vi "Static Test.vi"(5 "Mechanical Zero":dbl, 9 "read buffer":string) -> (4 "Elbow Angle (deg)":dbl, 6 "Goniometer\nAngle Raw":dynamicdata(graph), 8 "Static LF":dbl, 10 "Static Load Force":dynamicdata(graph), 14 "Grip Force":dynamicdata(graph), 15 "GF":dbl)   [LabVIEW 2018]
doc: "VI for GF and LF conversion."
panel:
  out "Dynamic Load Force":dbl
  # "\"Throw away\" data"
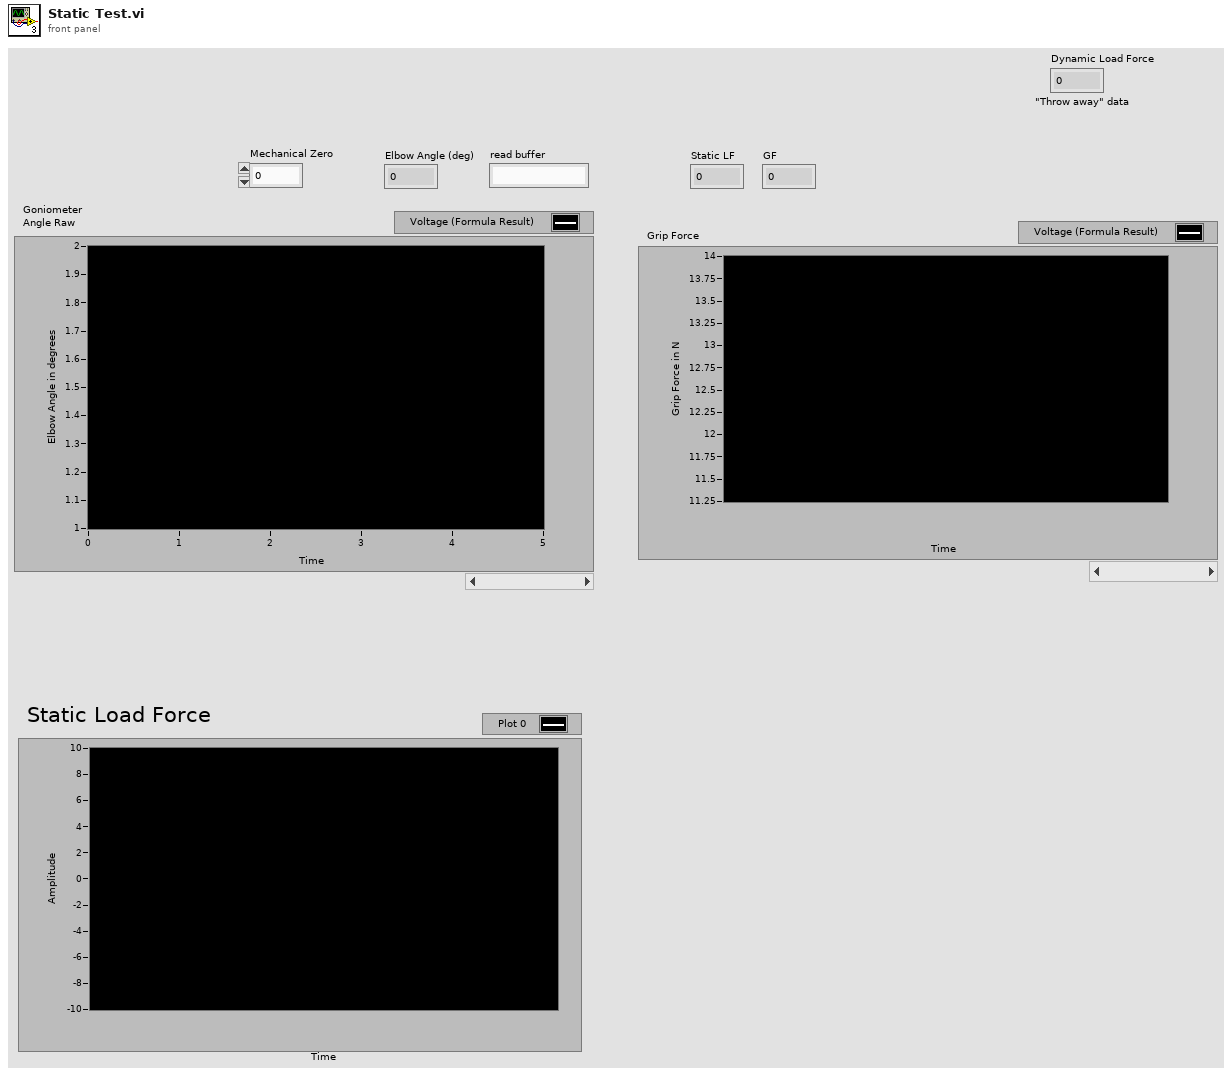
[diagram p1: front panel]
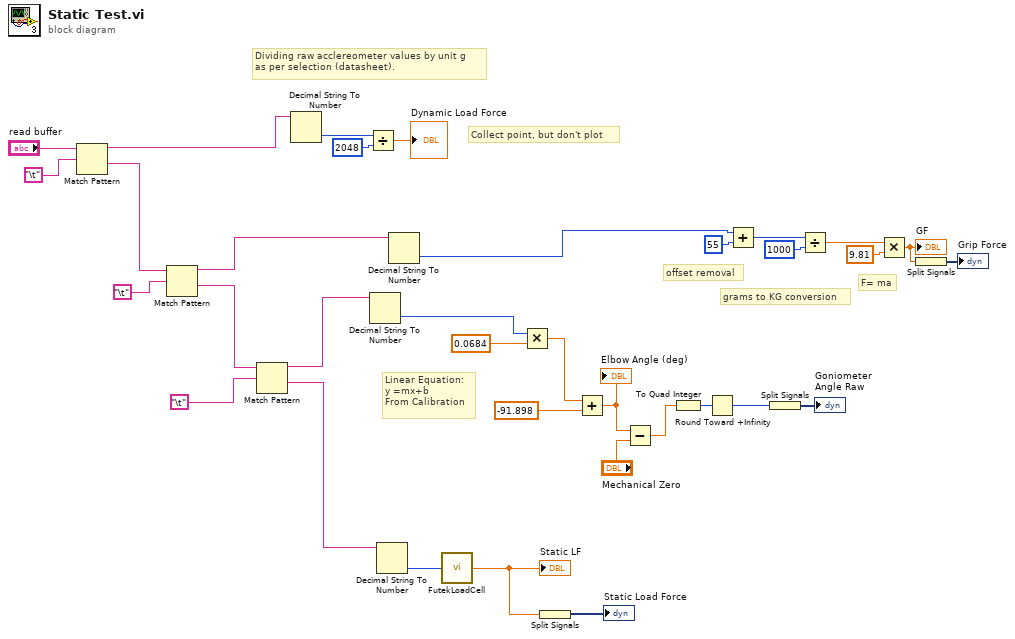
[diagram p0: block diagram]
diagram:
  # "Collect point, but don't plot"
  # "F= ma"
  # "offset removal"
  # "grams to KG conversion"
  # "Linear Equation:\ny =mx+b\nFrom Calibration"
  # "Dividing raw acclereometer values by unit g\nas per selection (datasheet)."
  n1 = Match Pattern(string="read buffer", regular expression="\t") -> (before substring=w34:string, after substring=w28:string)  [unwired: 1 in, 2 out]
  n2 = Match Pattern(string=w28, regular expression="\t") -> (before substring=w27:string, after substring=w16:string)  [unwired: 1 in, 2 out]
  n3 = Match Pattern(string=w16, regular expression="\t") -> (before substring=w15:string, after substring=w14:string)  [unwired: 1 in, 2 out]
  n4 = Decimal String To Number(string=w34) -> (number=w31:i32)  [unwired: 2 in, 1 out]
  n5 = Divide(x=w31, y=2048) -> (x/y=→"Dynamic Load Force":dbl)
  n6 = Decimal String To Number(string=w15) -> (number=w22:i32)  [unwired: 2 in, 1 out]
  n7 = Decimal String To Number(string=w14) -> (number=w2:i32)  [unwired: 2 in, 1 out]
  n8 = Decimal String To Number(string=w27) -> (number=w4:i32)  [unwired: 2 in, 1 out]
  n9 = call "FutekLoadCell.vi"("Futek Sensor Reading"=w2) -> ("Futek Force"=w1:dbl)
  "Static LF" <- w1
  n10 = Multiply(x=w22, y=0.0684 ("x")) -> (x*y=w25:dbl)
  n11 = Split Signals(w1) -> (→"Static Load Force":dynamicdata)  [unwired: 1 in]
  n12 = Add(x=w25, y=-91.898 ("x")) -> (x+y=w20:dbl)
  "Elbow Angle (deg)" <- w20
  n13 = Subtract(x=w20, y="Mechanical Zero") -> (x-y=w21:dbl)
  n14 = To Quad Integer(1:w21) -> (0:w18:i64)
  n15 = Round Toward +Infinity(x=w18) -> (ceil(x): smallest int >= x=w17:i64)
  n16 = Add(x=w4, y=55) -> (x+y=w10:i32)
  n17 = Split Signals(w17) -> (→"Goniometer\nAngle Raw":dynamicdata)  [unwired: 1 in]
  n18 = Divide(x=w10, y=1000) -> (x/y=w7:dbl)
  n19 = Multiply(x=w7, y=9.81) -> (x*y=w11:dbl)
  "GF" <- w11
  n20 = Split Signals(w11) -> (→"Grip Force":dynamicdata)  [unwired: 1 in]
